vi "Get State (uSMC) array.vi"(8 "error in":errorcluster, 11 "Visa array in":refnum<visa-resource-name>[](array[refnum])) -> (0 "error out":errorcluster, 2 "Array":T1[](array[typedef]), 3 "Visa array out":refnum<visa-resource-name>[](array[refnum]))   [LabVIEW 2010, in "SignalWriterMH110203USBStepperMotor.lvclass"]
uses:
  SignalWriterMH110203USBStepperMotor.lvclass
  Get State Control (uSMC).ctl
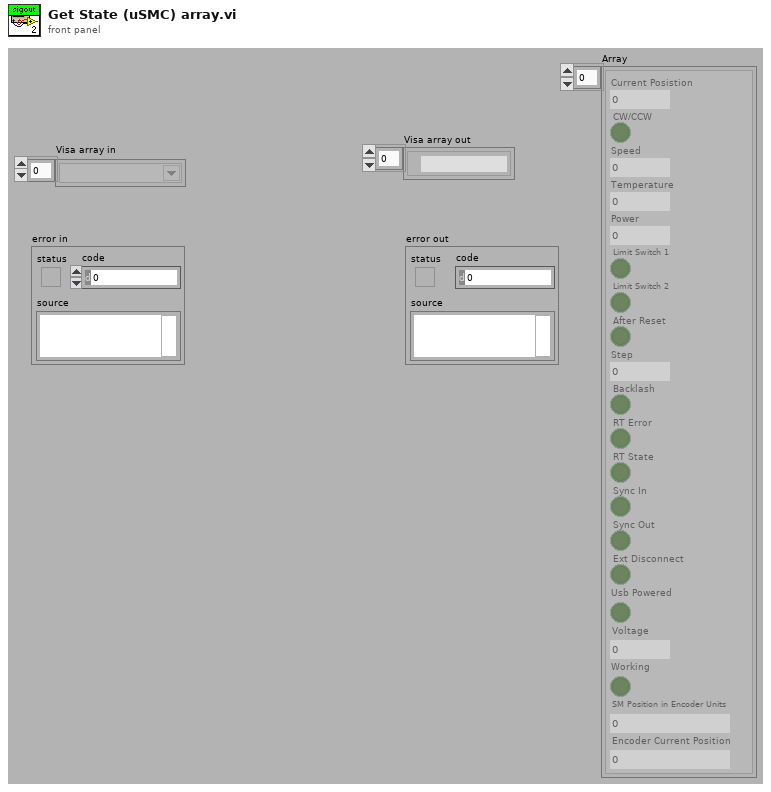
[diagram p1: front panel]
types:
  T1 = typedef "SignalWriterMH110203USBStepperMotor.lvclass/Get State Control (uSMC).ctl" = cluster{"Current Posistion":dbl, "CW/CCW":bool, "Speed":u16, "Temperature":dbl, "Power":u16, "Limit Switch 1":bool, "Limit Switch 2":bool, "After Reset":bool, "Step":u8, "Backlash":bool, "RT Error":bool, "RT State":bool, "Sync In":bool, "Sync Out":bool, "Ext Disconnect":bool, "Usb Powered":bool, "Voltage":dbl, "Working":bool, "SM Position in Encoder Units":i32, "Encoder Current Position":i32}
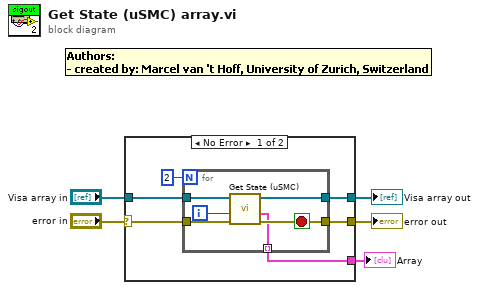
[diagram p0: block diagram]
diagram:
  n1 = case shown="No Error" "error in" {
    selector: "error in" -> [w7 w19]
    tunnel: [w11 w19] -> w5
    tunnel: "Visa array in" -> [w9 w18]
    tunnel: [w8 w18] -> w3
    tunnel: [w6 _] -> w1
    frame No Error {
      n2 = for {
        N: 2 -> [_]
        tunnel: [w17] -> w11
        tunnel: w7 -> [w16]
        tunnel: [w14] -> w8
        tunnel: w9 -> [w13]
        tunnel: [w12] -> w6 mode=indexing
        i -> [w15]
        stop <- w17 stop-if-true
        n3 = call "Get State (uSMC).vi"("error in (no error)"=w16, "SM number"=w15, "Visa array in"=w13) -> ("error out"=w17:errorcluster, "State cluster"=w12:T1, "Visa array out"=w14:refnum<visa-resource-name>[])  [unwired: 6 in]
      }
    }
    frame Error {
    }
  }
  "error out" <- w5
  "Visa array out" <- w3
  "Array" <- w1
